vi "MakeAcqusitionPath.vi"(9 "Comment to current acquisition (f.e. \"25ml_H2O\")":string, 10 "Acquisition title (main folder name)":string, 11 "Path":path=path "C:/Data") -> (0 "error out":errorcluster, 3 "Acqusition path":path)   [LabVIEW 2016]
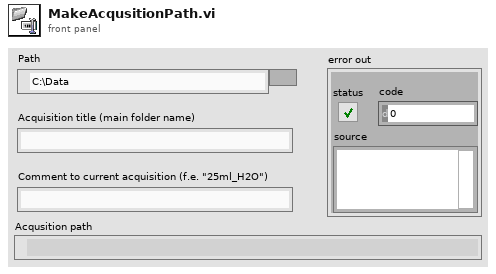
[diagram p1: front panel]
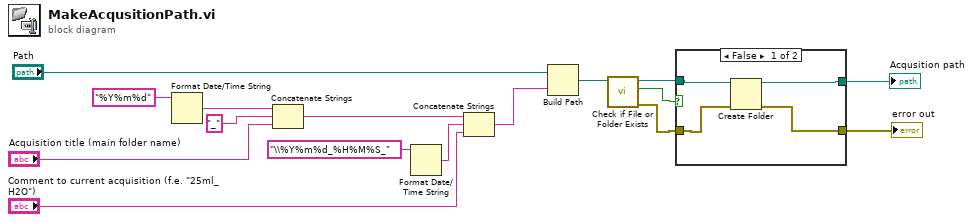
[diagram p0: block diagram]
diagram:
  n1 = Format Date/Time String(time format string (%c)="%Y%m%d") -> (date/time string=w3:string)  [unwired: 2 in]
  n2 = Concatenate Strings(w3, "_" ("string"), "Acquisition title (main folder name)") -> (w7:string)
  n3 = Format Date/Time String(time format string (%c)="\\%Y%m%d_%H%M%S_") -> (date/time string=w8:string)  [unwired: 2 in]
  n4 = Concatenate Strings(w7, w8, "Comment to current acquisition (f.e. \"25ml_H2O\")") -> (w10:string)
  n5 = Build Path(base path="Path", name or relative path=w10) -> (appended path=w11:path)
  n6 = call <vilib>:"Check if File or Folder Exists.vi"("path"=w11) -> ("error out"=w14:errorcluster, "file or folder exists?"=w12:bool, "dup path"=w13:path)  [unwired: 8 in]
  n7 = case shown="False" w12 {
    tunnel: [w17 w22] -> w15
    tunnel: w13 -> [w20 w22]
    tunnel: w14 -> [w19 w21]
    tunnel: [w18 w21] -> w16
    frame False {
      n8 = Create Folder(path (use dialog)=w20, error in=w19) -> (created path=w17:path, error out=w18:errorcluster)  [unwired: 1 in, 1 out]
    }
    frame True {
    }
  }
  "Acqusition path" <- w15
  "error out" <- w16
